vi "SEH Error Processor.vi"(4 "Valid Default":bool, 6 "Default Action":T1={"Number of Retries"=0, "Output Classification"="", "Retry"=FALSE, "Classify Output"=FALSE, "Classify Notification"=FALSE, "Notification Classification"="", "Convert Output to Warning"=FALSE, "Clear Output"=FALSE, "Notify"=FALSE, "Priority"=0, "Detect Warning"=FALSE, "Call VI"=FALSE, "VI to Call"="*Non-critical*"}, 8 "Error to Check":errorcluster, 9 "Detect Any Warnings":bool, 10 "Iteration":i32, 11 "Error Handling Info":T2[](array[typedef])) -> (0 "error out":errorcluster, 1 "Loop?":bool, 2 "Classification":string, 5 "Internal Error":errorcluster)   [LabVIEW 2017]
doc: "This SubVI exists so that changes made to the underlying error handling code will propagate to existing instances of the Express VI."
uses:
  <vilib>/NI/SEH/Controls/SEH/SEH Error Options.ctl
  <vilib>/NI/SEH/Controls/SEH/SEH Shared Error Options.ctl
  <userlib>/_SEH/Controls/Shared/SEH Error Notification Command.ctl
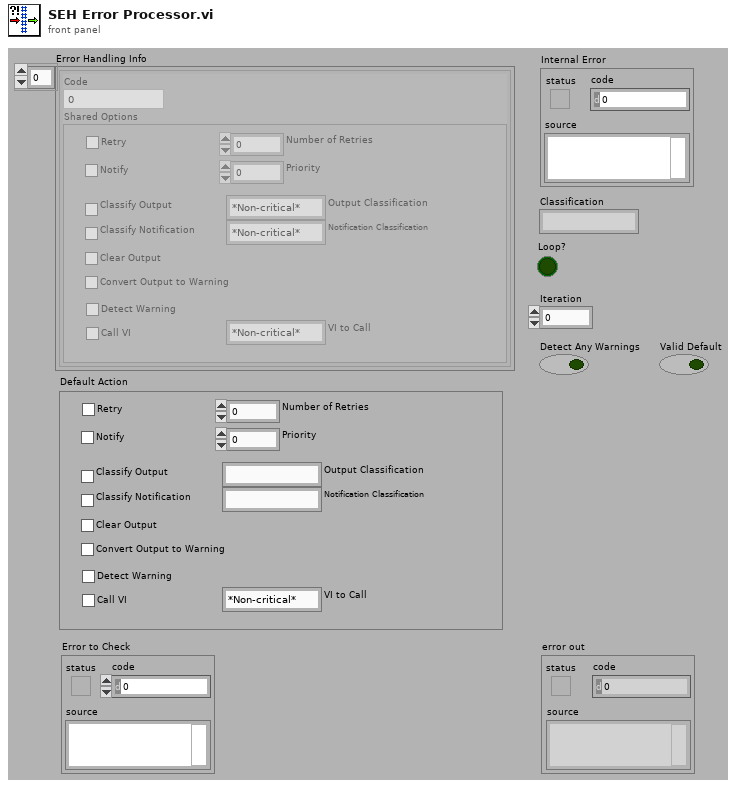
[diagram p1: front panel]
types:
  T1 = typedef "SEH Shared Error Options.ctl" = cluster{"Number of Retries":i32, "Output Classification":string, "Retry":bool, "Classify Output":bool, "Classify Notification":bool, "Notification Classification":string, "Convert Output to Warning":bool, "Clear Output":bool, "Notify":bool, "Priority":i32, "Detect Warning":bool, "Call VI":bool, "VI to Call":string}
  T2 = typedef "SEH Error Options.ctl" = cluster{"Code":i32, "Shared Options":T1}
  T3 = typedef "SEH Error Notification Command.ctl" = enum16{"Init", "Send Error", "Check Error", "Invalid Command"}
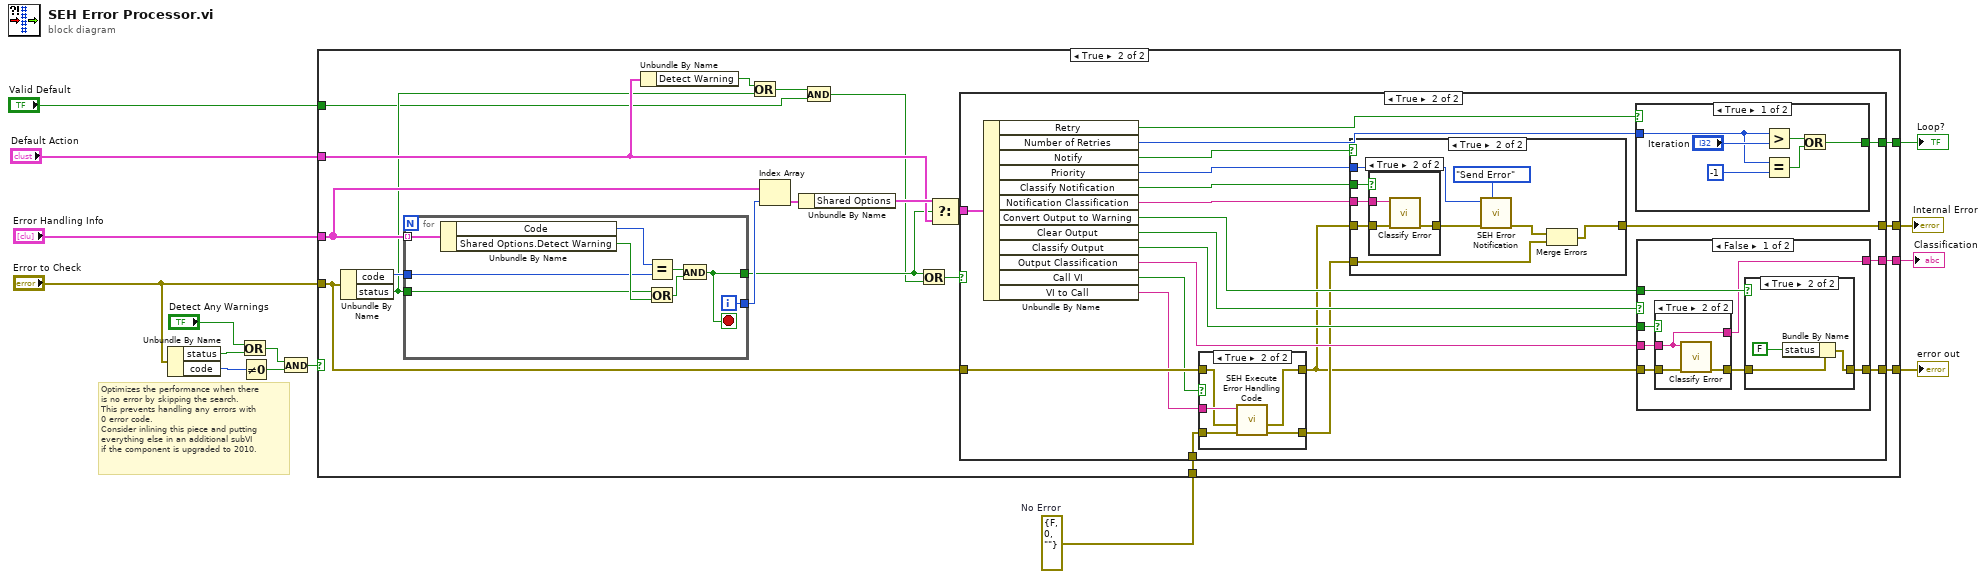
[diagram p0: block diagram]
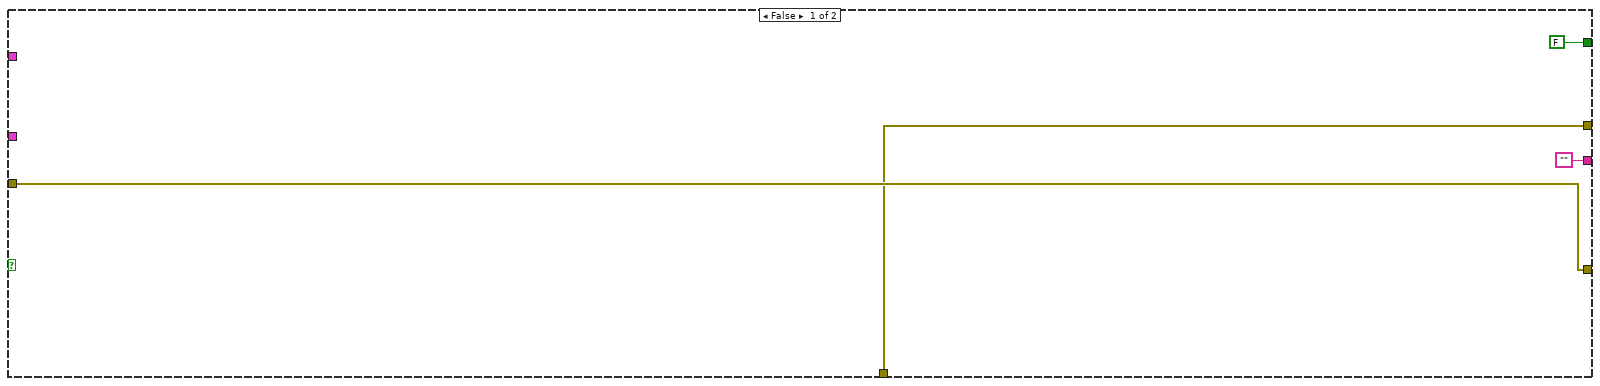
[diagram p2: hidden frame]
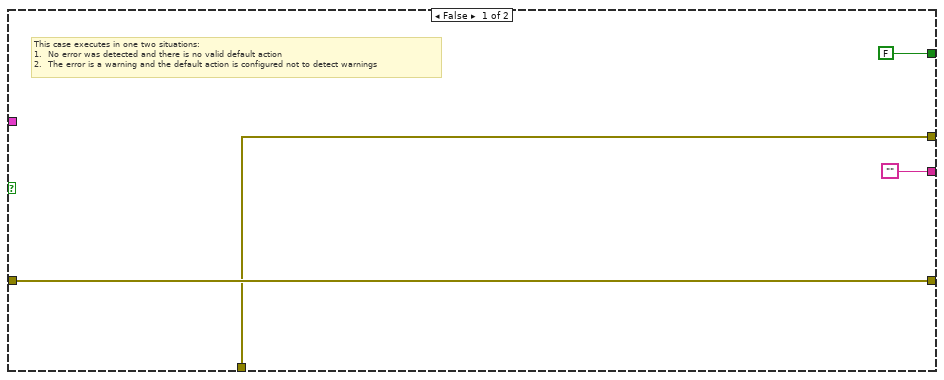
[diagram p3: hidden frame]
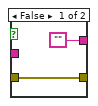
[diagram p8: hidden frame]
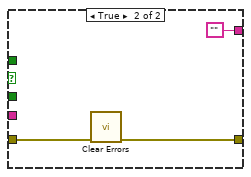
[diagram p9: hidden frame]
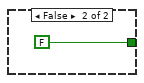
[diagram p10: hidden frame]
diagram:
  w1 = errorcluster {"status"=FALSE, "code"=0, "source"=""}  # No Error
  # "Optimizes the performance when there\nis no error by skipping the search.\nThis prevents handling any errors with\n0 error code.\nConsider inlining this piece and putting \neverything else in an additional subVI \nif the component is upgraded to 2010."
  n1 = Unbundle By Name("Error to Check") -> ("status"=w8:bool, "code"=w11:i32)
  n2 = Or(x="Detect Any Warnings", y=w8) -> (x .or. y?=w7:bool)
  n3 = Not Equal To 0?(x=w11) -> (x != 0?=w10:bool)
  n4 = And(x=w7, y=w10) -> (x .and. y?=w9:bool)
  n5 = case shown="True" w9 {
    tunnel: "Error Handling Info" -> [_ w39]
    tunnel: "Error to Check" -> [w19 w34]
    tunnel: [w19 w38] -> w14
    tunnel: [FALSE ("T button?") w37] -> w13
    tunnel: "Default Action" -> [_ w30]
    tunnel: "Valid Default" -> [_ w26]
    tunnel: ["" w22] -> w3
    tunnel: [w16 w21] -> w2
    tunnel: w1 -> [w16 w20]
    frame False {
    }
    frame True {
      n6 = Unbundle By Name(w34) -> ("code"=w33:i32, "status"=w28:bool)
      n7 = for {
        tunnel: w39 -> [w48] mode=indexing
        tunnel: [w44] -> w25
        tunnel: [w46] -> w36
        tunnel: w33 -> [w41]
        tunnel: w28 -> [w40]
        i -> [w46]
        stop <- w44 stop-if-true
        n8 = Unbundle By Name(w48) -> ("Code"=w45:i32, "Shared Options.Detect Warning"=w42:bool)
        n9 = Equal?(x=w45, y=w41) -> (x = y?=w47:bool)
        n10 = Or(x=w40, y=w42) -> (x .or. y?=w43:bool)
        n11 = And(x=w47, y=w43) -> (x .and. y?=w44:bool)
      }
      n12 = Unbundle By Name(w30) -> ("Detect Warning"=w29:bool)
      n13 = Or(x=w29, y=w28) -> (x .or. y?=w27:bool)
      n14 = Index Array(array=w39, index=w36) -> (element=w35:T2)
      n15 = Unbundle By Name(w35) -> ("Shared Options"=w32:T1)
      n16 = And(x=w27, y=w26) -> (x .and. y?=w24:bool)
      n17 = Or(x=w25, y=w24) -> (x .or. y?=w23:bool)
      n18 = Select(t=w32, s=w25, f=w30) -> (s? t:f=w31:T1)
      n19 = case shown="True" w23 {
        tunnel: [FALSE ("T button?") w73] -> w37
        tunnel: w34 -> [w51 w59]
        tunnel: [w51 w72] -> w38
        tunnel: w31 -> [_ w69]
        tunnel: ["" w60] -> w22
        tunnel: [w49 w56] -> w21
        tunnel: w20 -> [w49 w55]
        frame False {
          # "This case executes in one two situations:\n1.  No error was detected and there is no valid default action\n2.  The error is a warning and the default action is configured not to detect warnings"
        }
        frame True {
          n20 = Unbundle By Name(w69) -> ("Retry"=w71:bool, "Number of Retries"=w70:i32, "Notify"=w68:bool, "Priority"=w67:i32, "Classify Notification"=w66:bool, "Notification Classification"=w65:string, "Convert Output to Warning"=w61:bool, "Clear Output"=w64:bool, "Classify Output"=w63:bool, "Output Classification"=w62:string, "Call VI"=w58:bool, "VI to Call"=w57:string)
          n21 = case shown="True" w58 {
            tunnel: w59 -> [w75 w79]
            tunnel: [w75 w78] -> w53
            tunnel: w57 -> [_ w80]
            tunnel: w55 -> [w74 w77]
            tunnel: [w74 w76] -> w54
            frame False {
            }
            frame True {
              n22 = call <userlib>:"SEH Execute Error Handling Code.vi"("Internal Error In"=w77, "Error to Process In"=w79, "Code to Execute"=w80) -> ("Internal Error Out"=w76:errorcluster, "Error to Process Out"=w78:errorcluster)  [unwired: 7 in]
            }
          }
          n23 = case shown="True" w68 {
            tunnel: w67 -> [_ w85]
            tunnel: w53 -> [_ w87]
            tunnel: w66 -> [_ w89]
            tunnel: w65 -> [_ w88]
            tunnel: [w81 w82] -> w56
            tunnel: w54 -> [w81 w83]
            frame False {
            }
            frame True {
              n24 = case shown="True" w89 {
                tunnel: w88 -> [_ w94]
                tunnel: w87 -> [w91 w93]
                tunnel: [w91 w92] -> w86
                frame False {
                }
                frame True {
                  n25 = call <vilib>:"Classify Error.vi"("Error to Classify"=w93, "String"=w94) -> ("Classified Error"=w92:errorcluster)  [unwired: 9 in]
                }
              }
              n26 = call <userlib>:"SEH Error Notification.vi"("Command"=SEH_Error_Notification_Command."Send Error", "Error to Send"=w86, "Priority"=w85) -> ("Transmission Error"=w84:errorcluster)  [unwired: 3 in, 5 out]
              n27 = Merge Errors(w84, w83) -> (w82:errorcluster)
            }
          }
          n28 = case shown="True" w71 {
            tunnel: [w114 FALSE] -> w73
            tunnel: w70 -> [w115 _]
            frame True {
              n29 = Greater?(x=w115, y="Iteration") -> (0:w119:bool)
              n30 = Equal?(x=w115, y=-1) -> (x = y?=w118:bool)
              n31 = Or(x=w119, y=w118) -> (x .or. y?=w114:bool)
            }
            frame False {
            }
          }
          n32 = case shown="False" w64 {
            tunnel: w53 -> [w99 w113]
            tunnel: [w97 w112] -> w72
            tunnel: w63 -> [w101 _]
            tunnel: w62 -> [w100 _]
            tunnel: w61 -> [w96 _]
            tunnel: [w95 ""] -> w60
            frame False {
              n33 = case shown="True" w101 {
                tunnel: w100 -> [_ w108]
                tunnel: w99 -> [w107 w110]
                tunnel: [w107 w109] -> w98
                tunnel: ["" w108] -> w95
                frame False {
                }
                frame True {
                  n34 = call <vilib>:"Classify Error.vi"("Error to Classify"=w110, "String"=w108) -> ("Classified Error"=w109:errorcluster)  [unwired: 9 in]
                }
              }
              n35 = case shown="True" w96 {
                tunnel: w98 -> [w102 w105]
                tunnel: [w102 w104] -> w97
                frame False {
                }
                frame True {
                  n36 = Bundle By Name(cluster=w105, "status"=FALSE) -> (w104:errorcluster)
                }
              }
            }
            frame True {
              n37 = call <vilib>:"Clear Errors.vi"("error in (no error)"=w113) -> ("error out"=w112:errorcluster)  [unwired: 1 in, 5 out]
            }
          }
        }
      }
    }
  }
  "error out" <- w14
  "Loop?" <- w13
  "Classification" <- w3
  "Internal Error" <- w2
